vi "Doppler_V1.6_dll.vi"(8 "error in (no error)":errorcluster, 9 "period":dbl, 10 "input cluster":T1, 11 "Data_complex":dbl[][](array[numeric])) -> (0 "error out":errorcluster, 3 "velocity_profile":dbl[][](graph))   [LabVIEW 2019]
uses:
  SD_OCT_DLL_Ver1.6.dll
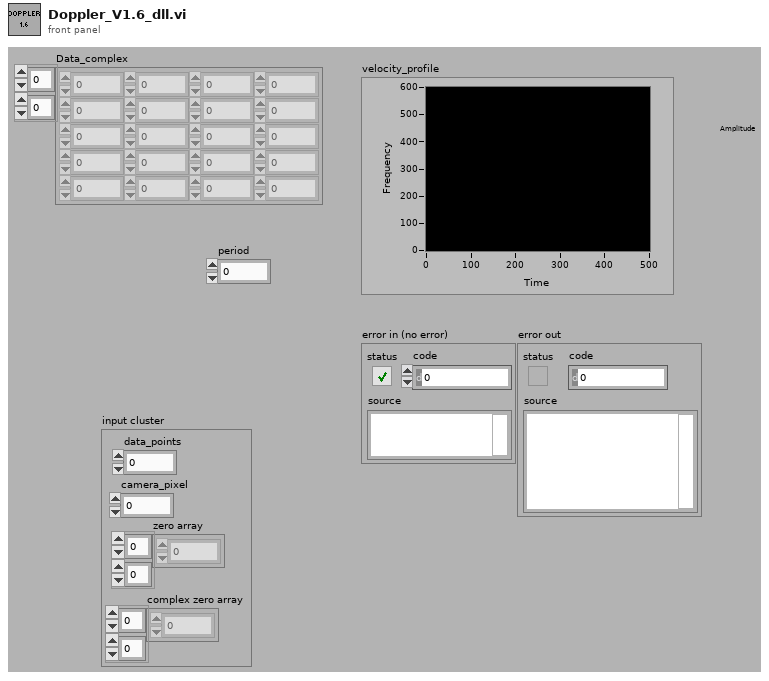
[diagram p1: front panel]
types:
  T1 = cluster{"data_points":i32, "camera_pixel":i32, "zero array":dbl[][], "complex zero array":dbl[][]}
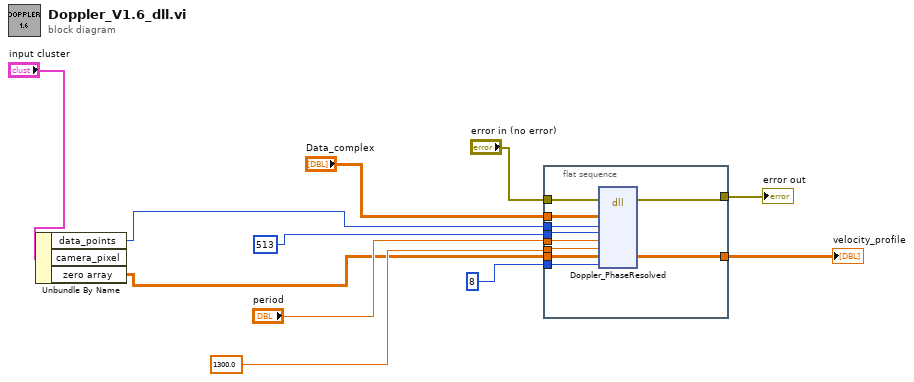
[diagram p0: block diagram]
diagram:
  n1 = Unbundle By Name("input cluster") -> ("data_points"=w5:i32, "zero array"=w4:dbl[][])  [unwired: 1 out]
  n2 = flat-sequence {
    tunnel: [w21] -> w11
    tunnel: "error in (no error)" -> [w20]
    tunnel: "Data_complex" -> [w19]
    tunnel: w5 -> [w18]
    tunnel: "period" -> [w17]
    tunnel: 1300.0 ("lambda") -> [w16]
    tunnel: [w15] -> w6
    tunnel: 8 ("core_number") -> [w14]
    tunnel: w4 -> [w13]
    tunnel: 513 ("camera_pixel") -> [w12]
    frame #0 {
      n3 = dll-call lib="C:/Users/hesfandi/Desktop/labview/LabViewCode/SD_OCT_DLL_Ver1.6.dll" fn="Doppler_PhaseResolved"(error in=w20, "Data_complex"=w19, "data_points"=w18, "camera_pixel"=w12, "period"=w17, "lambda"=w16, "velocity_profile"=w13, "core_number"=w14) -> (error out=w21:errorcluster, "velocity_profile"=w15:dbl[][])  [unwired: 9 in, 1 out]
    }
  }
  "error out" <- w11
  "velocity_profile" <- w6
